vi "uSubscription Create.vi"(8 "error in (no error)":errorcluster, 10 "Topics":string[](array[string]), 11 "uClient_Subscriber":refnum<class "uClient_Subscriber.lvclass">) -> (0 "error out":errorcluster, 2 "Filtered Topics":string[](array[string]), 3 "uSubscriptions out":refnum<class "uSubscription.lvclass">[](array[class]))   [LabVIEW 2021, in "uFramework.lvlib" / "uSubscription.lvclass"]
doc: "Pass in a list of topics and get subscriptions for the topics that conform to the subscription policy."
uses:
  uSubscription.lvclass
  uClient_Subscriber/uClient_Subscriber.lvclass
  U:/Projects/LABME/Src/uFramework/uClient/uClient.lvclass
  uClient/uClient.lvclass/uClient.ctl
  uClient_Subscriber/uClient_Subscriber.lvclass/uClient_Subscriber.ctl
  uPolicy/uPolicy.lvclass/uPolicy.ctl
  uSubscription.lvclass/uSubscription.ctl
  uPolicy/Read uNotifyMode.vi
  uPolicy/Read uStringManipulation.vi
  uTransport/uTransport.lvclass
  uPolicy/uPolicy.lvclass
  uNotifyMode/uNotifyMode.lvclass
  uStringManipulation/uStringManipulation.lvclass
  uClient/uClient.lvclass
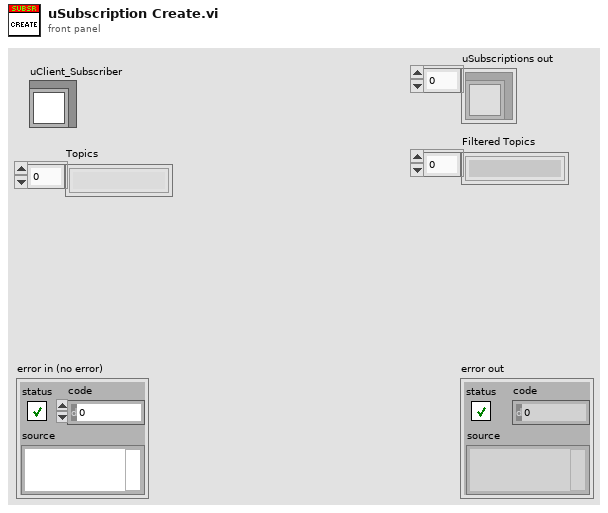
[diagram p1: front panel]
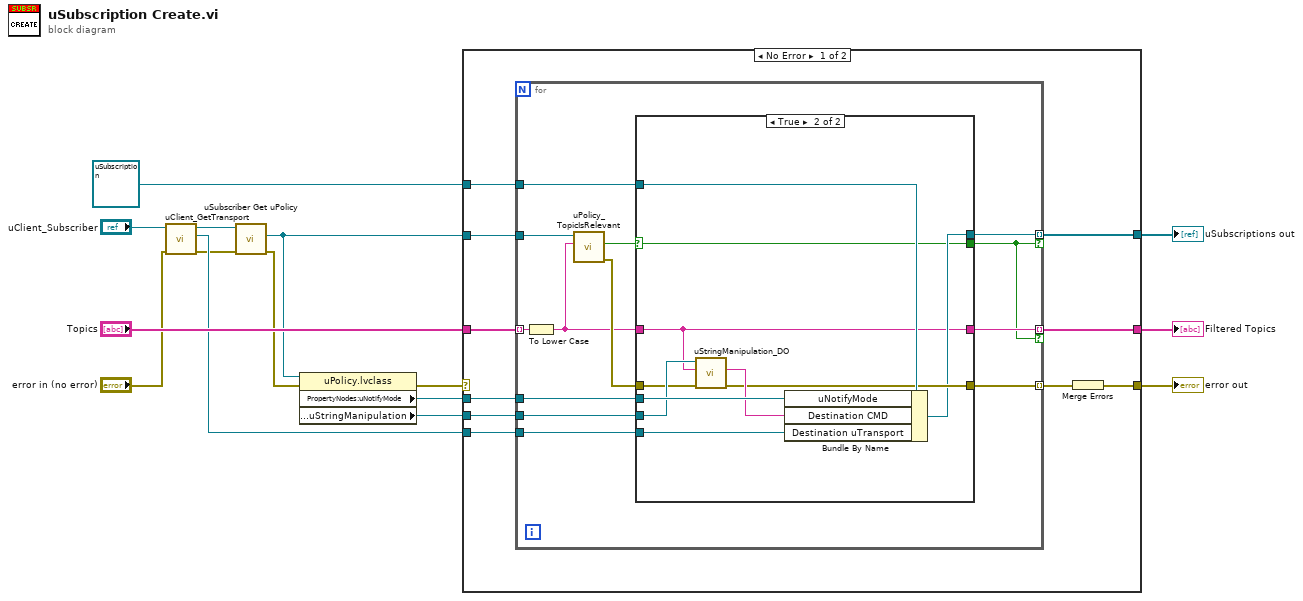
[diagram p0: block diagram]
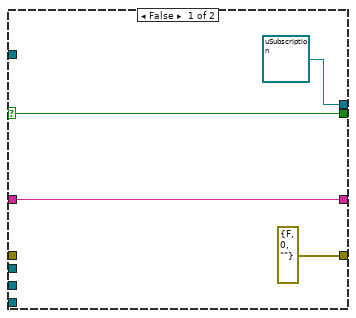
[diagram p2: hidden frame]
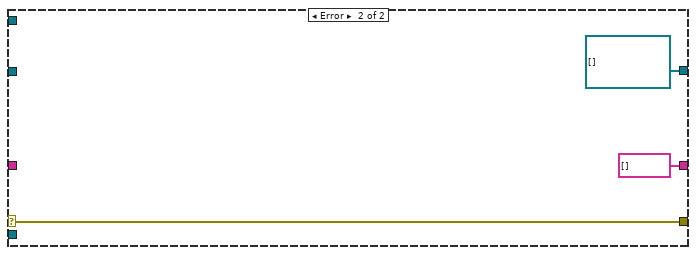
[diagram p3: hidden frame]
diagram:
  n1 = call "uClient_GetTransport.vi"("error in (no error)"="error in (no error)", "uClient in"="uClient_Subscriber") -> ("error out"=w4:errorcluster, "uTransport"=w6:refnum<class "uTransport.lvclass">, "uClient out"=w5:refnum<class "uClient_Subscriber.lvclass">)  [unwired: 7 in]
  n2 = call "uSubscriber Get uPolicy.vi"("error in (no error)"=w4, "uClient_Subscriber in"=w5) -> ("error out"=w3:errorcluster, "uPolicy"=w2:refnum<class "uPolicy.lvclass">)  [unwired: 7 in, 1 out]
  n3 = property class="uPolicy.lvclass"(reference=w2, error in=w3) -> (error out=w10:errorcluster, "PropertyNodes:uNotifyMode"=w11:refnum<class "uNotifyMode.lvclass">, "PropertyNodes:uStringManipulation"=w12:refnum<class "uStringManipulation.lvclass">)  [unwired: 1 out]
  n4 = case shown="No Error" w10 {
    selector: w10 -> [_ w55]
    tunnel: refnum<class "uSubscription.lvclass"> refnum ("uSubscription in") -> [w25 _]
    tunnel: "Topics" -> [w24 _]
    tunnel: [w19 w55] -> w13
    tunnel: w12 -> [w23 _]
    tunnel: w11 -> [w22 _]
    tunnel: w2 -> [w21 _]
    tunnel: [w18 refnum<class "uSubscription.lvclass">[] []] -> w9
    tunnel: w6 -> [w17 _]
    tunnel: [w16 string[] []] -> w1
    frame No Error {
      n5 = for {
        tunnel: w25 -> [w38]
        tunnel: w24 -> [w35] mode=indexing
        tunnel: w23 -> [w34]
        tunnel: w22 -> [w37]
        tunnel: w21 -> [w36]
        tunnel: [w33] -> w20 mode=indexing
        tunnel: [w30] -> w18 mode=indexing if=w27
        tunnel: w17 -> [w29]
        tunnel: [w28] -> w16 mode=indexing if=w27
        n6 = To Lower Case(string=w35) -> (all lower case string=w26:string)
        n7 = call-dynamic "uPolicy_TopicIsRelevant.vi"("Observed Topic (Lower Case)"=w26, "uPolicy_All in"=w36) -> ("error out"=w31:errorcluster, "Relevant?"=w32:bool)  [unwired: 7 in, 1 out]
        n8 = case shown="True" w32 {
          selector: w32 -> [w40 w45]
          tunnel: w38 -> [_ w52]
          tunnel: w37 -> [_ w51]
          tunnel: w26 -> [w39 w43]
          tunnel: w34 -> [_ w49]
          tunnel: [errorcluster {"status"=FALSE, "code"=0, "source"=""} ("error out") w48] -> w33
          tunnel: w31 -> [_ w47]
          tunnel: [refnum<class "uSubscription.lvclass"> refnum ("uSubscription in") w46] -> w30
          tunnel: [w40 w45] -> w27
          tunnel: w29 -> [_ w44]
          tunnel: [w39 w43] -> w28
          frame False {
          }
          frame True {
            n9 = call-dynamic "uStringManipulation_DO.vi"("error in (no error)"=w47, "String in"=w43, "uStringManipulation in"=w49) -> ("error out"=w48:errorcluster, "String"=w50:string)  [unwired: 6 in, 1 out]
            n10 = Bundle By Name(cluster=w52, "uNotifyMode"=w51, "Destination CMD"=w50, "Destination uTransport"=w44) -> (w46:refnum<class "uSubscription.lvclass">)
          }
        }
      }
      n11 = Merge Errors(w20) -> (w19:errorcluster)
    }
    frame Error {
    }
  }
  "error out" <- w13
  "uSubscriptions out" <- w9
  "Filtered Topics" <- w1
